vi "UMLEditor RemoveAggregationAttributes.vi"(1 "StartEndNodes":T1, 5 "error in (no error)":errorcluster) -> (15 "NodeModified":refnum<class "AbstractNode.lvclass">, 16 "Modified?":bool, 19 "error out":errorcluster)   [LabVIEW 2020]
doc: "Gets current diagram values"
uses:
  <resource>/Framework/Providers/Open_GDS/UML/AbstractNode_class/AbstractNode.lvclass
  <resource>/Framework/Providers/Open_GDS/UML/ClassNode_class/ExternalSetTypes.ctl
  <resource>/Framework/Providers/Open_GDS/UML/ClassNode_class/ClassNode.lvclass
  C:/Program Files (x86)/National Instruments/LabVIEW 2020/resource/Framework/Providers/Open_GDS/UML/AbstractNode_class/AbstractNode.lvclass
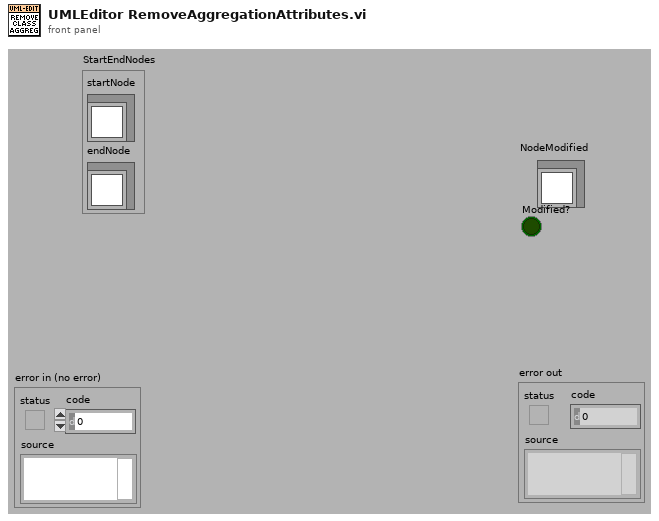
[diagram p1: front panel]
types:
  T1 = cluster{"startNode":refnum<class "AbstractNode.lvclass">, "endNode":refnum<class "AbstractNode.lvclass">}
  T2 = typedef "ClassNode.lvclass/ExternalSetTypes.ctl" = enum16{"Name", "Attributes", "Methods", "Position", "ShowMethods", "ShowAttributes", "ClassPath"}
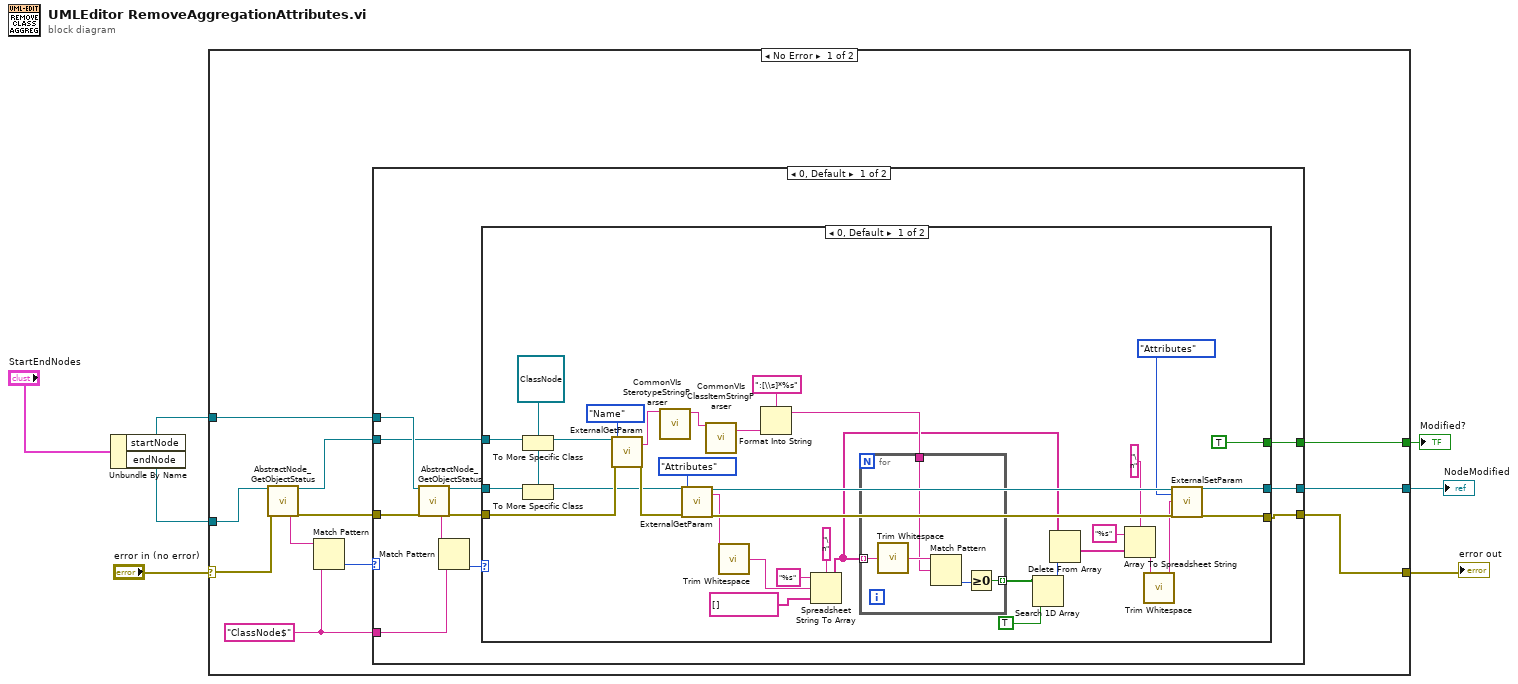
[diagram p0: block diagram]
diagram:
  n1 = Unbundle By Name("StartEndNodes") -> ("startNode"=w2:refnum<class "AbstractNode.lvclass">, "endNode"=w1:refnum<class "AbstractNode.lvclass">)
  n2 = case shown="No Error" "error in (no error)" {
    selector: "error in (no error)" -> [w9 w71]
    tunnel: [w14 w71] -> w6
    tunnel: [w12 _] -> w5
    tunnel: [w11 _] -> w4
    tunnel: w1 -> [w10 _]
    tunnel: w2 -> [w8 _]
    frame No Error {
      w17 = "ClassNode$" ("regular expression")
      n3 = call <resource>:"AbstractNode_GetObjectStatus.vi"("reference in"=w10, "error in (no error)"=w9) -> ("Class name"=w18:string, "reference out"=w13:refnum<class "AbstractNode.lvclass">, "error out"=w15:errorcluster)  [unwired: 15 out]
      n4 = Match Pattern(string=w18, regular expression=w17) -> (offset past match=w16:i32)  [unwired: 4 out]
      n5 = case shown="0, Default" w16 {
        tunnel: w8 -> [w25 _]
        tunnel: w17 -> [w24 _]
        tunnel: w15 -> [w22 w70]
        tunnel: [w23 w70] -> w14
        tunnel: w13 -> [w21 _]
        tunnel: [w20 _] -> w12
        tunnel: [w19 _] -> w11
        frame 0, Default {
          n6 = call <resource>:"AbstractNode_GetObjectStatus.vi"("reference in"=w25, "error in (no error)"=w22) -> ("Class name"=w29:string, "reference out"=w26:refnum<class "AbstractNode.lvclass">, "error out"=w27:errorcluster)  [unwired: 15 out]
          n7 = Match Pattern(string=w29, regular expression=w24) -> (offset past match=w28:i32)  [unwired: 4 out]
          n8 = case shown="0, Default" w28 {
            tunnel: w27 -> [w57 w69]
            tunnel: w26 -> [w32 _]
            tunnel: [w59 w69] -> w23
            tunnel: w21 -> [w34 _]
            tunnel: [w53 _] -> w20
            tunnel: [TRUE _] -> w19
            frame 0, Default {
              w30 = refnum<class "ClassNode.lvclass"> refnum ("reference")
              n9 = To More Specific Class(target class=w30, reference=w34) -> (specific class reference=w33:refnum<class "ClassNode.lvclass">)  [unwired: 1 in, 1 out]
              n10 = To More Specific Class(target class=w30, reference=w32) -> (specific class reference=w31:refnum<class "ClassNode.lvclass">)  [unwired: 1 in, 1 out]
              n11 = call <resource>:"ExternalGetParam.vi"("reference"=w33, "setParameter"=ExternalSetTypes."Name", "error in (no error)"=w57) -> ("string"=w55:string, "error out"=w56:errorcluster)  [unwired: 15 out]
              n12 = call <resource>:"CommonVIs SterotypeStringParser.vi"("SterotypeStringIn"=w55) -> ("Name"=w50:string)  [unwired: 18 out]
              n13 = call <resource>:"ExternalGetParam.vi"("reference"=w31, "setParameter"=ExternalSetTypes."Attributes", "error in (no error)"=w56) -> ("reference out"=w62:refnum<class "ClassNode.lvclass">, "string"=w51:string, "error out"=w61:errorcluster)  [unwired: 14 out]
              n14 = call <resource>:"CommonVIs ClassItemStringParser.vi"("ClassItemNameIn"=w50) -> ("Name"=w49:string)  [unwired: 18 out]
              n15 = call <vilib>:"Trim Whitespace.vi"("string"=w51) -> ("trimmed string"=w48:string)  [unwired: 1 in]
              n16 = Format Into String(format string=":[\\s]*%s", w49) -> (resulting string=w44:string)  [unwired: 2 in, 1 out]
              n17 = Spreadsheet String To Array(delimiter (Tab)="\n", format string="%s", spreadsheet string=w48, array type (2D Dbl)=string[] []) -> (array=w41:string[])
              n18 = for {
                tunnel: w41 -> [w68] mode=indexing
                tunnel: w44 -> [w66]
                tunnel: [w64] -> w43 mode=indexing
                n19 = call <vilib>:"Trim Whitespace.vi"("string"=w68) -> ("trimmed string"=w67:string)  [unwired: 1 in]
                n20 = Match Pattern(string=w67, regular expression=w66) -> (offset past match=w65:i32)  [unwired: 4 out]
                n21 = Greater Or Equal To 0?(x=w65) -> (x >= 0?=w64:bool)
              }
              n22 = Search 1D Array(1D array=w43, element=TRUE) -> (index of element=w40:i32)  [unwired: 1 out]
              n23 = Delete From Array(array=w41, index=w40) -> (array with subset deleted=w39:string[])  [unwired: 1 in, 1 out]
              n24 = Array To Spreadsheet String(delimiter (Tab)="\n", array=w39, 3:"%s" ("format string")) -> (spreadsheet string=w36:string)
              n25 = call <vilib>:"Trim Whitespace.vi"("string"=w36) -> ("trimmed string"=w35:string)  [unwired: 1 in]
              n26 = call-dynamic "ExternalSetParam.vi"("reference"=w62, "setParameter"=ExternalSetTypes."Attributes", "string"=w35, "error in (no error)"=w61) -> ("reference out"=w53:refnum<class "ClassNode.lvclass">, "error out"=w59:errorcluster)  [unwired: 14 in]
            }
            frame -1 {
            }
          }
        }
        frame -1 {
        }
      }
    }
    frame Error {
    }
  }
  "error out" <- w6
  "NodeModified" <- w5
  "Modified?" <- w4
